vi "SOUR_POW_CORR_COLL_BSEN_RCF.vi"(0 "VISA IN":refnum<visa-resource-name>, 5 "error in":errorcluster, 7 "Channel":i32) -> (14 "VISA Out":refnum<visa-resource-name>, 16 "Data":string, 19 "error out":errorcluster)   [LabVIEW 2018, in "PNA-X.lvlib"]
doc: "SOURce:POWer:CORRection:COLLect:BSENsor:RCFactor? \nReturn Type Numeric \nDefault 100 \nSOURce<cnum>:POWer:CORRection:COLLect:<pmChan>SENsor:SELect \n(Read-Write) Sets and returns the power sensor channel (A or B) to be used. This performs the same \nfunction as the Use this sensor only checkbox in the Power Sensor Settings dialog. \nNote: This write portion of this command is only necessary when performing an SMC calibration. \nParameters \n<cnum> Any existing channel number. If unspecified, value is set to 1 \n<pmChan> Power Meter channel. Choose from: \nA - Channel A \nB - Channel B \nExamples SOUR:POW:CORR:COLL:<pmChan>SEN:SEL 'Write \nsource1:power2:correction:collect:bsensor:select? 1e9 'Read \nQuery Syntax SOURce:POWer:CORRection:COLLect:ASENsor:SELect? <Frequency>"
uses:
  PNA-X.lvlib
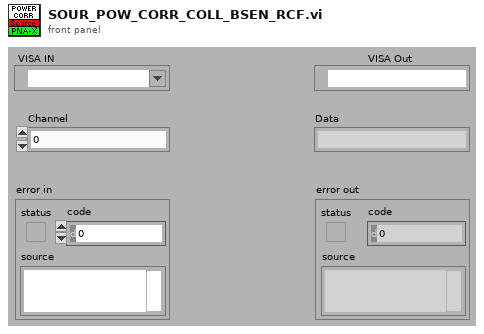
[diagram p1: front panel]
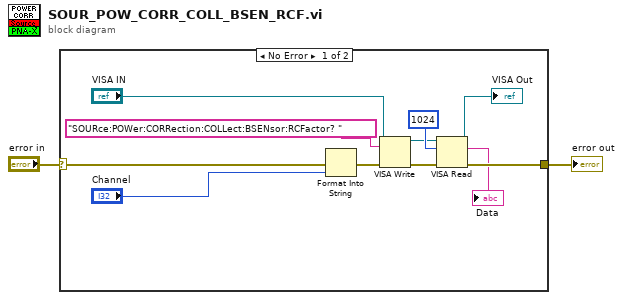
[diagram p0: block diagram]
diagram:
  n1 = case shown="No Error" "error in" {
    selector: "error in" -> [w13 w14]
    tunnel: [w7 w14] -> w1
    frame No Error {
      n2 = Format Into String(error in=w13, "Channel") -> (error out=w12:errorcluster)  [unwired: 2 in, 1 out]
      n3 = VISA Write(VISA resource name="VISA IN", write buffer="SOURce:POWer:CORRection:COLLect:BSENsor:RCFactor? " ("Cmdline"), error in (no error)=w12) -> (VISA resource name out=w8:refnum<visa-resource-name>, error out=w10:errorcluster)  [unwired: 1 out]
      n4 = VISA Read(VISA resource name=w8, byte count=1024, error in (no error)=w10) -> (VISA resource name out=→"VISA Out":refnum<visa-resource-name>, read buffer=→"Data":string, error out=w7:errorcluster)  [unwired: 1 out]
    }
    frame Error {
    }
  }
  "error out" <- w1
